vi "IR Laser Diode Controller.vi"() -> ()   [LabVIEW 2014]
doc: "This example shows how to use the TL4000 series driver package with different TL4000 devices (ITC4xxx, LDC4xxx, TED4xxx or CLD1xxx).\n\nNote:\nParts of the Front Panel will be disabled and grayed out if the connected device doesn't suppport the associated functions."
uses:
  <instrlib>/TL4000/TL4000.llb/z_StateMachineTypeDef.ctl
panel:
  out "TEC on?":bool
  out "LD on?":bool
  in  "Config Button":bool
  in  "TEC Button":bool
  in  "LD Button":bool
  in  "Quit Button":bool
  out "PD Optical Power":dbl caption="PD Optical Power [W]" format="%#_4g"
  out "PD Current":dbl caption="PD Current [mA]" format="%#.4g"
  out "Temperature":dbl caption="Temperature [°C]" format="%.2f"
  in  "Temperature Setpoint":dbl=25.0 caption="Temperature [°C]" min=10.0 max=50.0 format="%.2f"
  in  "LD Current Setpoint":dbl caption="LD Current [A]" min=0.0 max=0.48 step=0.1 format="%.4g"
  out "TEC Power":dbl caption="TEC Power [W]" format="%.4f"
  out "TEC Voltage":dbl caption="TEC Voltage [V]" format="%.4f"
  out "TEC Current":dbl caption="TEC Current [A]" format="%.4f"
  out "LD Power":dbl caption="LD electr. Power [W]" format="%.4f"
  out "LD Voltage":dbl caption="LD Voltage [V]" format="%.4f"
  out "LD Current":dbl caption="LD Current [A]" format="%.4f"
  out "Serial Number":string
  out "Device Name":string
  out "Manufacturer Name":string
  out "Firmware Revision":string
  in  "Tab Control":enum32{"Page 1", "Page 2"}(tab)
  in  "error in":errorcluster
  out "error out":errorcluster
  in  "Handle":refnum<visa-resource-name>
  out "State100":T1 caption="States"
  out "user event out":refnum<user-event>
  out "Connected":bool
  in  "Device Type":T2(ring)
  out "Status Bar":string
  # "TL4000 Series Example"
  # "Setpoints:"
  # "Measurement:"
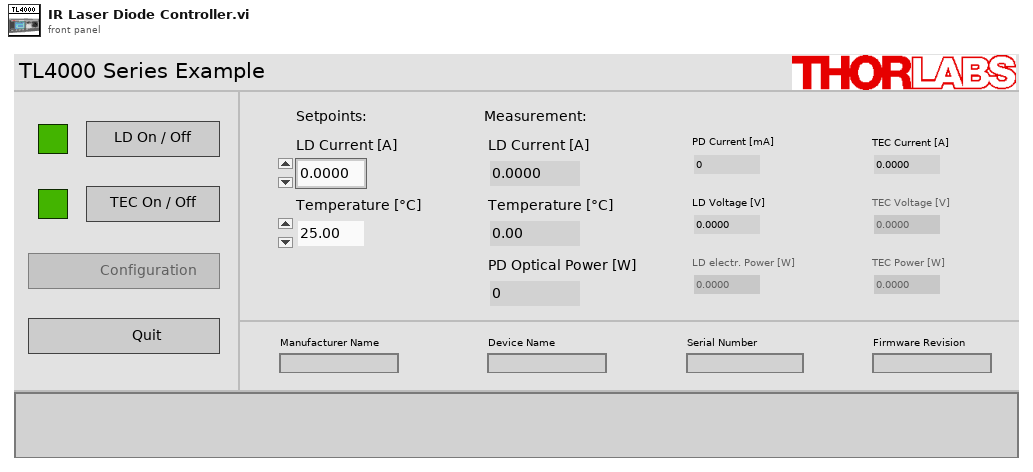
[diagram p1: front panel]
types:
  T1 = typedef "z_StateMachineTypeDef.ctl" = enum16{"Initialize", "1", "2", "3", "4", "5", "6", "7", "8", "9", "10", "15", "20", "25", "30", "35", "40", "45", "50", "55", "59", "60", "65", "70", "75", "76", "77", "78", "79", "80", "85", "90", "91", "92", "93", "94", "95", "96", "97", "98", "99", "100", "105", "110", "120", "130", "140", "150", "160", "170", "180", "190", "200", "205", "210", "215", "220", "230", "240", "245", "250", "255", "260", "270", "280", "290", "300", "310", "313", "315", "318", "320", "330", "340", "350", "360", "370", "380", "390", "400", "410", "420", "430", "440", "450", "460", "470", "480", "490", "500", "510", "520", "523", "525", "528", "530", "540", "550", "560", "570", "580", "590", "600", "605", "610", "620", "630", "640", "650", "660", "670", "680", "690", "700", "710", "720", "730", "740", "750", "760", "770", "780", "790", "800", "810", "820", "830", "840", "850", "860", "870", "880", "890", "900", "910", "920", "930", "940", "950", "960", "970", "980", "990", "1000", "1010", "1020", "1030", "1040", "1050", "1060", "1070", "1080", "1090", "1100", "1110", "1120", "1130", "1140", "1150", "1160", "1170", "1180", "1190", "1200", "1210", "1220", "1230", "1240", "1250", "1260", "1270", "1280", "1290", "1300", "1310", "1320", "1330", "1340", "1350", "1360", "1370", "1380", "1390", "1400", "1410", "1420", "1430", "1440", "1450", "1460", "1470", "1480", "1490", "1500", "Fehler I", "Fehler II", "Fehler III", "Fehler IV", "Fehler V", "Fehler VI", "Fehler VII", "Fehler VIII", "Fehler IX", "Fehler X", "Stop"}
  T2 = enum16{"LDC4000", "CLD1000", "ITC4000", "TED4000"}
  T3 = enum8{"Enabled", "Disabled", "Disabled and Grayed Out"}
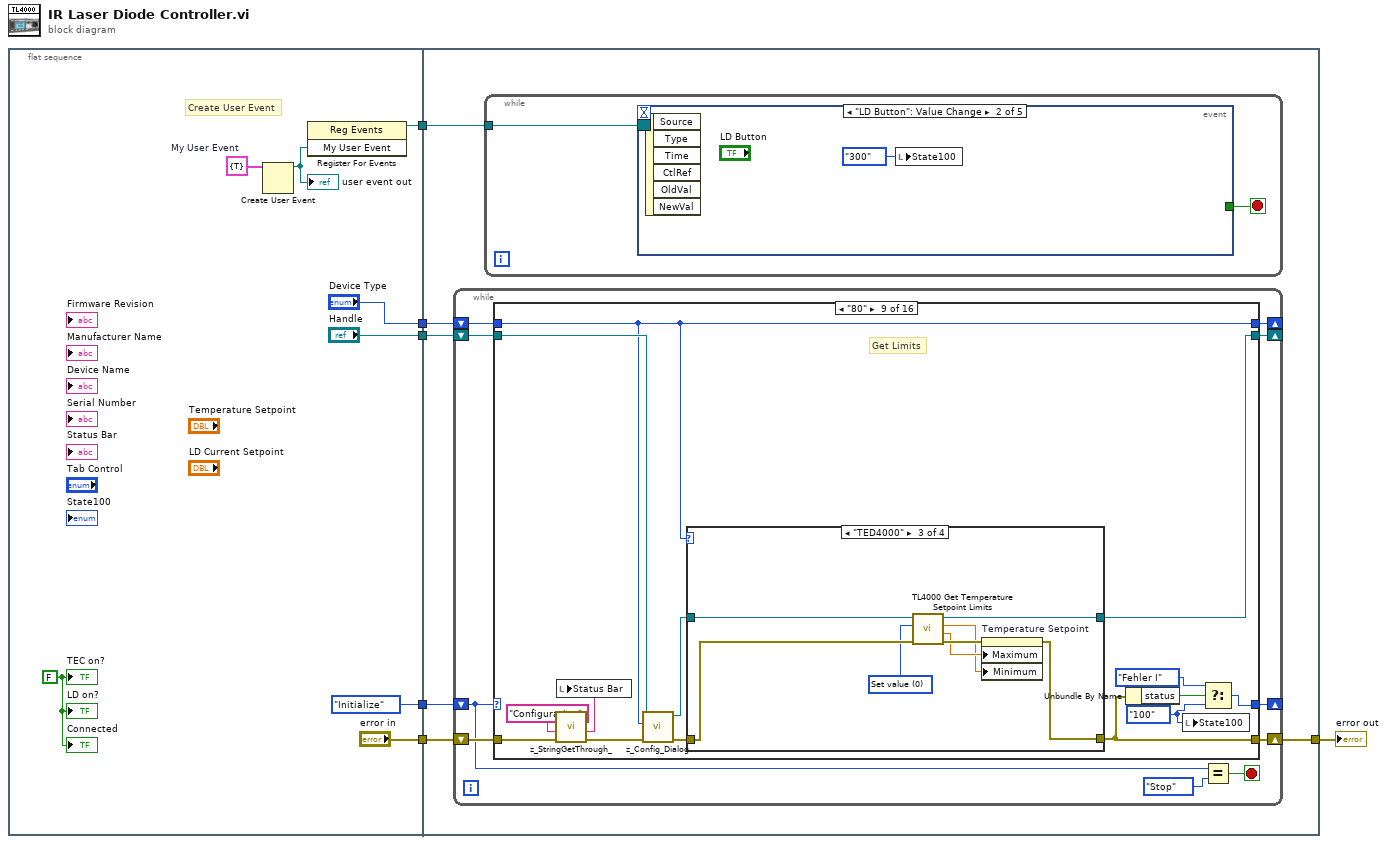
[diagram p0: block diagram]
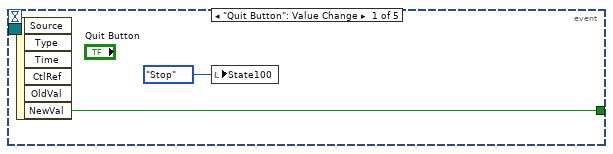
[diagram p2: hidden frame]
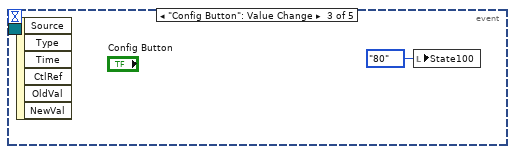
[diagram p3: hidden frame]
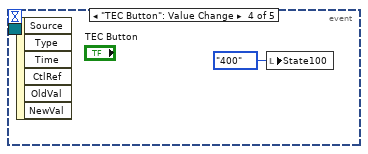
[diagram p4: hidden frame]
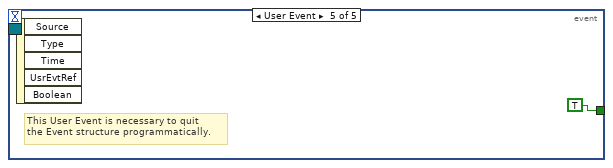
[diagram p5: hidden frame]
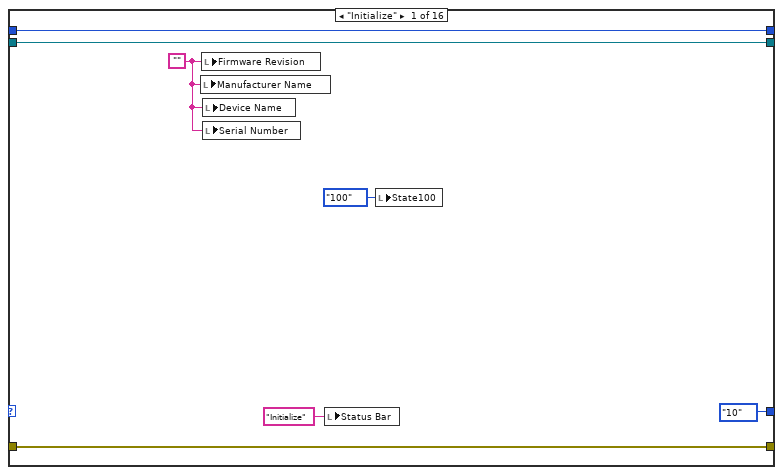
[diagram p6: hidden frame]
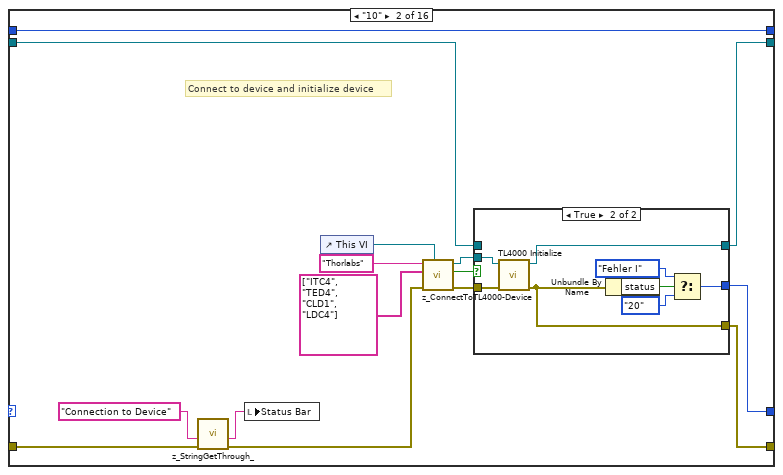
[diagram p7: hidden frame]
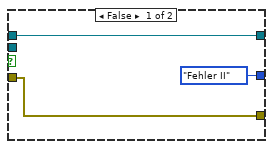
[diagram p8: hidden frame]
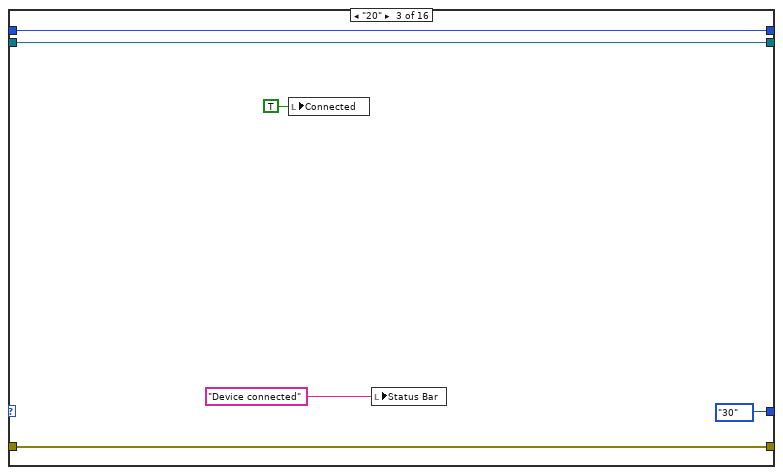
[diagram p9: hidden frame]
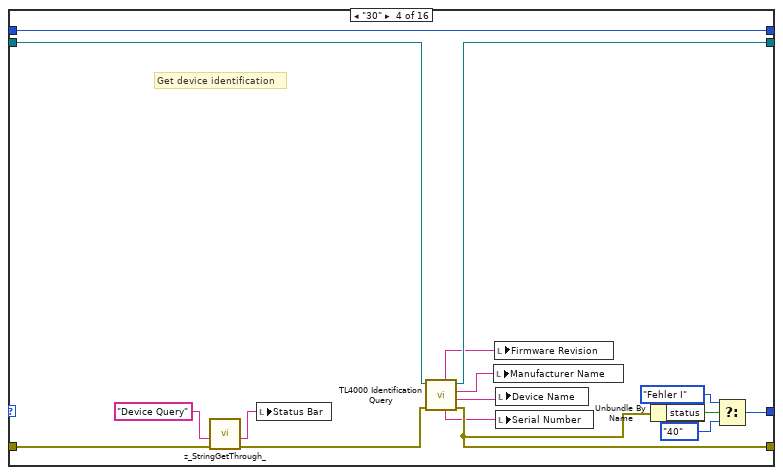
[diagram p10: hidden frame]
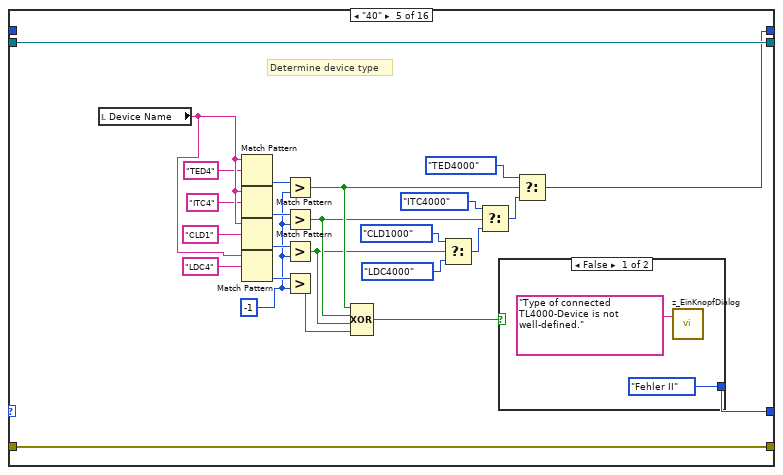
[diagram p11: hidden frame]
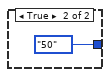
[diagram p12: hidden frame]
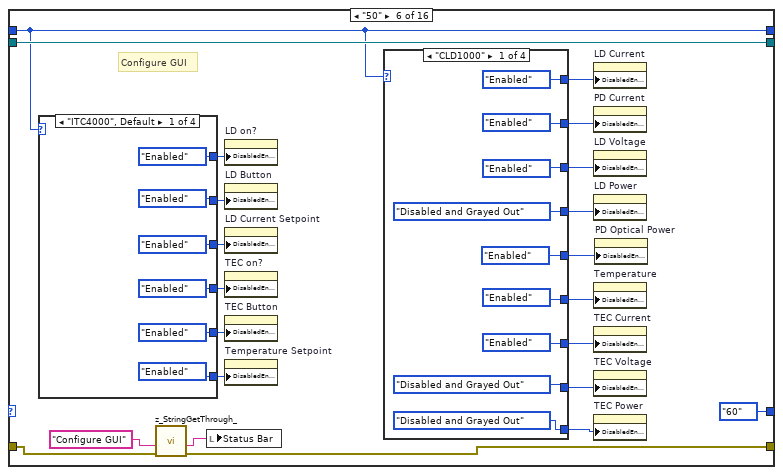
[diagram p13: hidden frame]
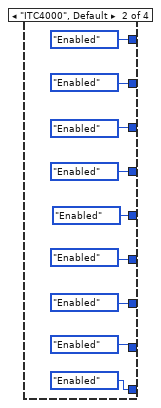
[diagram p14: hidden frame]
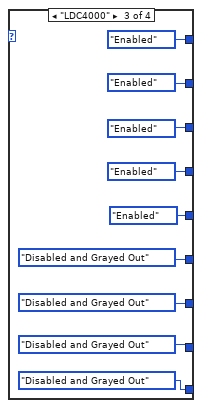
[diagram p15: hidden frame]
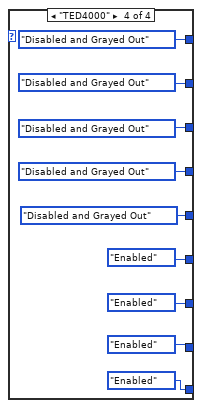
[diagram p16: hidden frame]
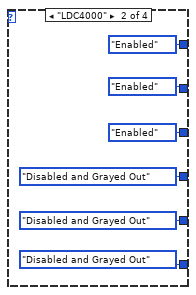
[diagram p17: hidden frame]
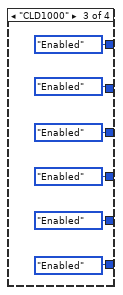
[diagram p18: hidden frame]
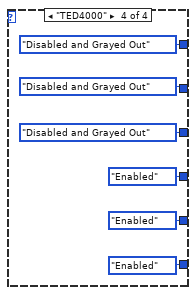
[diagram p19: hidden frame]
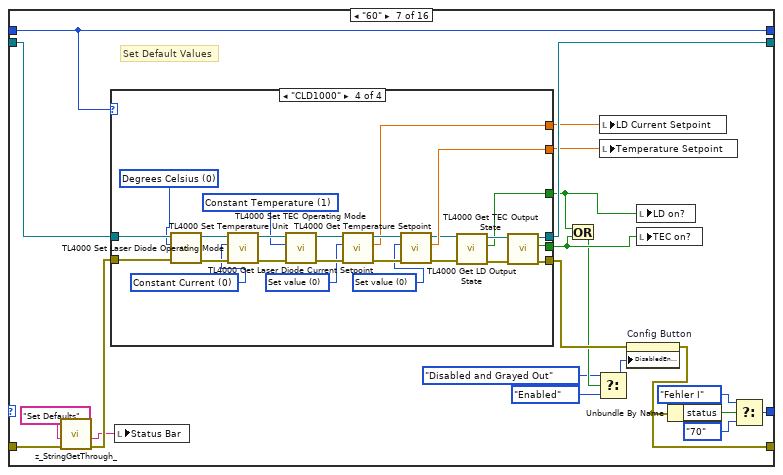
[diagram p20: hidden frame]
diagram:
  n1 = flat-sequence {
    tunnel: ["error in"] -> w6
    tunnel: ["Handle"] -> w4
    tunnel: ["Device Type"] -> w3
    tunnel: [z_StateMachineTypeDef."Initialize" ("States")] -> w2
    tunnel: [w8] -> w1
    tunnel: w6 -> [w20]
    tunnel: [w19] -> w5
    tunnel: w4 -> [w18]
    tunnel: w3 -> [w17]
    tunnel: w2 -> [w16]
    tunnel: w1 -> [w15]
    frame #0 {
      w10 = FALSE ("TEC on?")
      w14 = cluster{"Boolean":bool} {"Boolean"=TRUE}  # My User Event
      # "Create User Event"
      n2 = Create User Event(user event datatype=w14) -> (user event=w7:refnum<user-event>)  [unwired: 1 in, 1 out]
      "user event out" <- w7
      n3 = register-events(w7) -> (reference out=w8:refnum<event-registration>)  [unwired: 2 in, 1 out]
      "Connected" <- w10
      "TEC on?" <- w10
      "LD on?" <- w10
    }
    frame #1 {
      n4 = while {
        shift-right: [w38] -> _
        shift-left: w16 -> [w29]
        shift-right: [w34] -> w19
        shift-left: w20 -> [w35]
        shift-right: [w32] -> _
        shift-left: w18 -> [w33]
        shift-right: [w30] -> _
        shift-left: w17 -> [w31]
        stop <- w36 stop-if-true
        n5 = case shown="\"80\"" w29 {
          tunnel: [z_StateMachineTypeDef."10" ("States") w55 z_StateMachineTypeDef."30" ("States") w90 w101 z_StateMachineTypeDef."60" ("States") w224 w314 w472 z_StateMachineTypeDef."200" ("States") w540 w674 w693 z_StateMachineTypeDef."Fehler II" ("States") z_StateMachineTypeDef."Stop" ("States") z_StateMachineTypeDef."Stop" ("States")] -> w38
          tunnel: w35 -> [w42 w51 w75 w87 w102 w134 w215 w306 w462 w517 w529 w670 w690 w697 w706 w713]
          tunnel: [w42 w54 w75 w85 w102 w133 w210 w310 w467 w517 w537 w667 w678 w703 w706 w712] -> w34
          tunnel: w33 -> [w41 w53 w74 w84 w118 w142 w220 w309 w469 w518 w539 w671 w691 w701 w707 w716]
          tunnel: [w41 w52 w74 w83 w118 w142 w219 w308 w465 w518 w538 w672 w686 w702 w707 w716] -> w32
          tunnel: w31 -> [w39 w47 w72 w78 _ w131 w216 w307 w464 w514 w526 w665 w685 w698 w705 w711]
          tunnel: [w39 w47 w72 w78 w94 w131 w216 w307 w464 w514 w526 w665 w685 w698 w705 w711] -> w30
          frame "Initialize" {
            w43 = ""
            n6 = local write "Manufacturer Name"(w43) -> ()
            n7 = local write "Firmware Revision"(w43) -> ()
            n8 = local write "Device Name"(w43) -> ()
            n9 = local write "Serial Number"(w43) -> ()
            n10 = local write "Status Bar"("Initialize" ("Statuszeile")) -> ()
            n11 = local write "State100"(z_StateMachineTypeDef."100" ("State100")) -> ()
          }
          frame "10" {
            # "Connect to device and initialize device"
            n12 = call <instrlib>:"z_StringGetThrough_.vi"("Error In"=w51, "String In"="Connection to Device") -> ("Error Out"=w50:errorcluster, "String Out"=w49:string)  [unwired: 8 in]
            n13 = local write "Status Bar"(w49) -> ()
            n14 = control-ref of="This VI"() -> (w59:refnum<vi>)
            n15 = call <instrlib>:"z_ConnectToTL4000-Device.vi"("VI reference"=w59, "error in"=w50, "Models"=string[] ["ITC4", "TED4", "CLD1", "LDC4"], "Manufacturer"="Thorlabs") -> ("error out"=w56:errorcluster, "FoundUSB"=w58:bool, "USB Ref"=w57:refnum<visa-resource-name>)  [unwired: 5 in]
            n16 = case shown="True" w58 {
              tunnel: w57 -> [_ w65]
              tunnel: w56 -> [w62 w67]
              tunnel: [z_StateMachineTypeDef."Fehler II" ("f") w68] -> w55
              tunnel: [w62 w66] -> w54
              tunnel: [w63 w64] -> w52
              tunnel: w53 -> [w63 _]
              frame False {
              }
              frame True {
                n17 = call <instrlib>:"TL4000 Initialize.vi"("error in (no error)"=w67, "resource name"=w65) -> ("error out"=w66:errorcluster, "instrument handle out"=w64:refnum<visa-resource-name>)  [unwired: 8 in]
                n18 = Unbundle By Name(w66) -> ("status"=w69:bool)
                n19 = Select(t=z_StateMachineTypeDef."Fehler I" ("States"), s=w69, f=z_StateMachineTypeDef."20") -> (s? t:f=w68:T1)
              }
            }
          }
          frame "20" {
            n20 = local write "Connected"(TRUE ("Connected")) -> ()
            n21 = local write "Status Bar"("Device connected" ("String In")) -> ()
          }
          frame "30" {
            # "Get device identification"
            n22 = call <instrlib>:"z_StringGetThrough_.vi"("Error In"=w87, "String In"="Device Query") -> ("Error Out"=w86:errorcluster, "String Out"=w89:string)  [unwired: 8 in]
            n23 = local write "Status Bar"(w89) -> ()
            n24 = call <instrlib>:"TL4000 Identification Query.vi"("error in (no error)"=w86, "instrument handle"=w84) -> ("error out"=w85:errorcluster, "Device Name"=w80:string, "Manufacturer Name"=w81:string, "instrument handle out"=w83:refnum<visa-resource-name>, "Serial Number"=w79:string, "Firmware Revision"=w82:string)  [unwired: 4 in]
            n25 = local write "Manufacturer Name"(w81) -> ()
            n26 = local write "Firmware Revision"(w82) -> ()
            n27 = local write "Device Name"(w80) -> ()
            n28 = local write "Serial Number"(w79) -> ()
            n29 = Unbundle By Name(w85) -> ("status"=w91:bool)
            n30 = Select(t=z_StateMachineTypeDef."Fehler I" ("States"), s=w91, f=z_StateMachineTypeDef."40") -> (s? t:f=w90:T1)
          }
          frame "40" {
            w108 = -1 ("y")
            # "Determine device type"
            n31 = local read "Device Name"() -> (w117:string)
            n32 = Match Pattern(string=w117, regular expression="TED4") -> (offset past match=w112:i32)  [unwired: 1 in, 3 out]
            n33 = Match Pattern(string=w117, regular expression="ITC4") -> (offset past match=w111:i32)  [unwired: 1 in, 3 out]
            n34 = Match Pattern(string=w117, regular expression="CLD1") -> (offset past match=w110:i32)  [unwired: 1 in, 3 out]
            n35 = Match Pattern(string=w117, regular expression="LDC4") -> (offset past match=w109:i32)  [unwired: 1 in, 3 out]
            n36 = Greater?(x=w112, y=w108) -> (0:w107:bool)
            n37 = Greater?(x=w111, y=w108) -> (0:w106:bool)
            n38 = Greater?(x=w110, y=w108) -> (0:w105:bool)
            n39 = Greater?(x=w109, y=w108) -> (0:w104:bool)
            n40 = Compound Arithmetic op=XOR(w107, w106, w105, w104) -> (w103:bool)
            n41 = Select(t=T2."CLD1000" ("Device_Type"), s=w105, f=T2."LDC4000" ("Device_Type")) -> (s? t:f=w95:T2)
            n42 = Select(t=T2."ITC4000" ("Device_Type"), s=w106, f=w95) -> (s? t:f=w99:T2)
            n43 = case shown="False" w103 {
              tunnel: [z_StateMachineTypeDef."Fehler II" ("States") z_StateMachineTypeDef."50" ("f")] -> w101
              frame False {
                n44 = call <instrlib>:"z_EinKnopfDialog.vi"("Message"="Type of connected TL4000-Device is not well-defined.") -> ()  [unwired: 1 in, 1 out]
              }
              frame True {
              }
            }
            n45 = Select(t=T2."TED4000" ("Device_Type"), s=w107, f=w99) -> (s? t:f=w94:T2)
          }
          frame "50" {
            # "Configure GUI"
            n46 = case shown="\"ITC4000\", Default" w131 {
              tunnel: [T3."Enabled" ("Disabled") T3."Enabled" ("Disabled") T3."Enabled" ("Disabled") T3."Disabled and Grayed Out" ("Disabled")] -> w141
              tunnel: [T3."Enabled" ("Disabled") T3."Enabled" ("Disabled") T3."Enabled" ("Disabled") T3."Disabled and Grayed Out" ("Disabled")] -> w140
              tunnel: [T3."Enabled" ("Disabled") T3."Enabled" ("Disabled") T3."Enabled" ("Disabled") T3."Disabled and Grayed Out" ("Disabled")] -> w139
              tunnel: [T3."Enabled" ("Disabled") T3."Disabled and Grayed Out" ("Disabled") T3."Enabled" ("Disabled") T3."Enabled" ("Disabled")] -> w138
              tunnel: [T3."Enabled" ("Disabled") T3."Disabled and Grayed Out" ("Disabled") T3."Enabled" ("Disabled") T3."Enabled" ("Disabled")] -> w137
              tunnel: [T3."Enabled" ("Disabled") T3."Disabled and Grayed Out" ("Disabled") T3."Enabled" ("Disabled") T3."Enabled" ("Disabled")] -> w136
              frame "ITC4000", Default {
              }
              frame "LDC4000" {
              }
              frame "CLD1000" {
              }
              frame "TED4000" {
              }
            }
            n47 = call <instrlib>:"z_StringGetThrough_.vi"("Error In"=w134, "String In"="Configure GUI") -> ("Error Out"=w133:errorcluster, "String Out"=w132:string)  [unwired: 8 in]
            n48 = local write "Status Bar"(w132) -> ()
            n49 = property on="LD on?" class="Bool (strict)"("DisabledEnum"=w141) -> ()  [unwired: 2 in, 2 out]
            n50 = property on="LD Button" class="Bool"("DisabledEnum"=w140) -> ()  [unwired: 2 in, 2 out]
            n51 = property on="LD Current Setpoint" class="DigNum (strict)"("DisabledEnum"=w139) -> ()  [unwired: 2 in, 2 out]
            n52 = property on="TEC on?" class="Bool (strict)"("DisabledEnum"=w138) -> ()  [unwired: 2 in, 2 out]
            n53 = property on="TEC Button" class="Bool"("DisabledEnum"=w137) -> ()  [unwired: 2 in, 2 out]
            n54 = property on="Temperature Setpoint" class="DigNum (strict)"("DisabledEnum"=w136) -> ()  [unwired: 2 in, 2 out]
            n55 = case shown="\"CLD1000\"" w131 {
              tunnel: [T3."Enabled" ("Disabled") T3."Enabled" ("Disabled") T3."Enabled" ("Disabled") T3."Disabled and Grayed Out" ("Disabled")] -> w123
              tunnel: [T3."Enabled" ("Disabled") T3."Enabled" ("Disabled") T3."Enabled" ("Disabled") T3."Disabled and Grayed Out" ("Disabled")] -> w124
              tunnel: [T3."Disabled and Grayed Out" ("Disabled") T3."Enabled" ("Disabled") T3."Enabled" ("Disabled") T3."Disabled and Grayed Out" ("Disabled")] -> w125
              tunnel: [T3."Enabled" ("Disabled") T3."Enabled" ("Disabled") T3."Disabled and Grayed Out" ("Disabled") T3."Enabled" ("Disabled")] -> w126
              tunnel: [T3."Enabled" ("Disabled") T3."Enabled" ("Disabled") T3."Disabled and Grayed Out" ("Disabled") T3."Enabled" ("Disabled")] -> w127
              tunnel: [T3."Disabled and Grayed Out" ("Disabled") T3."Enabled" ("Disabled") T3."Disabled and Grayed Out" ("Disabled") T3."Enabled" ("Disabled")] -> w128
              tunnel: [T3."Disabled and Grayed Out" ("Disabled") T3."Enabled" ("Disabled") T3."Disabled and Grayed Out" ("Disabled") T3."Enabled" ("Disabled")] -> w130
              tunnel: [T3."Enabled" ("Disabled") T3."Enabled" ("Disabled") T3."Enabled" ("Disabled") T3."Disabled and Grayed Out" ("Disabled")] -> w129
              tunnel: [T3."Enabled" ("Disabled") T3."Enabled" ("Disabled") T3."Enabled" ("Disabled") T3."Disabled and Grayed Out" ("Disabled")] -> w122
              frame "CLD1000" {
              }
              frame "ITC4000", Default {
              }
              frame "LDC4000" {
              }
              frame "TED4000" {
              }
            }
            n56 = property on="LD Current" class="DigNum (strict)"("DisabledEnum"=w129) -> ()  [unwired: 2 in, 2 out]
            n57 = property on="PD Current" class="DigNum (strict)"("DisabledEnum"=w123) -> ()  [unwired: 2 in, 2 out]
            n58 = property on="LD Voltage" class="DigNum (strict)"("DisabledEnum"=w124) -> ()  [unwired: 2 in, 2 out]
            n59 = property on="LD Power" class="DigNum (strict)"("DisabledEnum"=w125) -> ()  [unwired: 2 in, 2 out]
            n60 = property on="Temperature" class="DigNum (strict)"("DisabledEnum"=w126) -> ()  [unwired: 2 in, 2 out]
            n61 = property on="TEC Current" class="DigNum (strict)"("DisabledEnum"=w127) -> ()  [unwired: 2 in, 2 out]
            n62 = property on="TEC Voltage" class="DigNum (strict)"("DisabledEnum"=w128) -> ()  [unwired: 2 in, 2 out]
            n63 = property on="TEC Power" class="DigNum (strict)"("DisabledEnum"=w130) -> ()  [unwired: 2 in, 2 out]
            n64 = property on="PD Optical Power" class="DigNum (strict)"("DisabledEnum"=w122) -> ()  [unwired: 2 in, 2 out]
          }
          frame "60" {
            # "Set Default Values"
            n65 = call <instrlib>:"z_StringGetThrough_.vi"("Error In"=w215, "String In"="Set Defaults") -> ("Error Out"=w214:errorcluster, "String Out"=w212:string)  [unwired: 8 in]
            n66 = case shown="\"CLD1000\"" w216 {
              tunnel: w214 -> [w249 w260 w280 w305]
              tunnel: [w232 w254 w276 w288] -> w211
              tunnel: w220 -> [w244 w261 w279 w300]
              tunnel: [w233 w255 w277 w289] -> w219
              tunnel: [w239 w263 0.0 ("Laser Diode Current Setpoint") w295] -> w218
              tunnel: [w238 0.0 ("Temperature Setpoint") w278 w294] -> w217
              tunnel: [w231 FALSE ("TEC Output") w275 w287] -> w208
              tunnel: [w230 w262 FALSE ("LD Output") w286] -> w209
              frame "ITC4000", Default {
                w225 = i16 0 items=["Set value", "Minimum value", "Maximum value"] ("Attribute (Set value)")
                w226 = i16 0 items=["Set value", "Minimum value", "Maximum value"] ("Attribute (Set value)")
                w227 = i16 1 items=["Constant Temperature"=1, "Current Source"=0] ("TEC Operating Mode (Constant Temperature)")
                w228 = i16 0 items=["Constant Current", "Constant Power"] ("Laser Diode Operating Mode (Constant Current)")
                w229 = i16 0 items=["Degrees Celsius", "Kelvin", "Degrees Fahrenheit"] ("Temperature Unit (Degrees Celsius)")
                n67 = call <instrlib>:"TL4000 Set Temperature Unit.vi"("error in (no error)"=w249, "Temperature Unit (Degrees Celsius)"=w229, "instrument handle"=w244) -> ("error out"=w248:errorcluster, "instrument handle out"=w243:refnum<visa-resource-name>)  [unwired: 7 in]
                n68 = call <instrlib>:"TL4000 Set Laser Diode Operating Mode.vi"("error in (no error)"=w248, "Laser Diode Operating Mode (Constant Current)"=w228, "instrument handle"=w243) -> ("error out"=w247:errorcluster, "instrument handle out"=w242:refnum<visa-resource-name>)  [unwired: 7 in]
                n69 = call <instrlib>:"TL4000 Set TEC Operating Mode.vi"("error in (no error)"=w247, "TEC Operating Mode (Constant Temperature)"=w227, "instrument handle"=w242) -> ("error out"=w246:errorcluster, "instrument handle out"=w241:refnum<visa-resource-name>)  [unwired: 7 in]
                n70 = call <instrlib>:"TL4000 Get Laser Diode Current Setpoint.vi"("error in (no error)"=w246, "Attribute (Set value)"=w226, "instrument handle"=w241) -> ("error out"=w245:errorcluster, "Laser Diode Current Setpoint"=w239:dbl, "instrument handle out"=w240:refnum<visa-resource-name>)  [unwired: 6 in]
                n71 = call <instrlib>:"TL4000 Get Temperature Setpoint.vi"("error in (no error)"=w245, "Attribute (Set value)"=w225, "instrument handle"=w240) -> ("error out"=w236:errorcluster, "Temperature Setpoint"=w238:dbl, "instrument handle out"=w237:refnum<visa-resource-name>)  [unwired: 6 in]
                n72 = call <instrlib>:"TL4000 Get LD Output State.vi"("error in (no error)"=w236, "instrument handle"=w237) -> ("error out"=w234:errorcluster, "LD Output"=w230:bool, "instrument handle out"=w235:refnum<visa-resource-name>)  [unwired: 7 in]
                n73 = call <instrlib>:"TL4000 Get TEC Output State.vi"("error in (no error)"=w234, "instrument handle"=w235) -> ("error out"=w232:errorcluster, "TEC Output"=w231:bool, "instrument handle out"=w233:refnum<visa-resource-name>)  [unwired: 7 in]
              }
              frame "LDC4000" {
                w250 = i16 0 items=["Set value", "Minimum value", "Maximum value"] ("Attribute (Set value)")
                w251 = i16 0 items=["Constant Current", "Constant Power"] ("Laser Diode Operating Mode (Constant Current)")
                n74 = call <instrlib>:"TL4000 Set Laser Diode Operating Mode.vi"("error in (no error)"=w260, "Laser Diode Operating Mode (Constant Current)"=w251, "instrument handle"=w261) -> ("error out"=w258:errorcluster, "instrument handle out"=w259:refnum<visa-resource-name>)  [unwired: 7 in]
                n75 = call <instrlib>:"TL4000 Get Laser Diode Current Setpoint.vi"("error in (no error)"=w258, "Attribute (Set value)"=w250, "instrument handle"=w259) -> ("error out"=w257:errorcluster, "Laser Diode Current Setpoint"=w263:dbl, "instrument handle out"=w256:refnum<visa-resource-name>)  [unwired: 6 in]
                n76 = call <instrlib>:"TL4000 Get LD Output State.vi"("error in (no error)"=w257, "instrument handle"=w256) -> ("error out"=w254:errorcluster, "LD Output"=w262:bool, "instrument handle out"=w255:refnum<visa-resource-name>)  [unwired: 7 in]
              }
              frame "TED4000" {
                w264 = i16 0 items=["Set value", "Minimum value", "Maximum value"] ("Attribute (Set value)")
                w265 = i16 1 items=["Constant Temperature"=1, "Current Source"=0] ("TEC Operating Mode (Constant Temperature)")
                w266 = i16 0 items=["Degrees Celsius", "Kelvin", "Degrees Fahrenheit"] ("Temperature Unit (Degrees Celsius)")
                n77 = call <instrlib>:"TL4000 Set Temperature Unit.vi"("error in (no error)"=w280, "Temperature Unit (Degrees Celsius)"=w266, "instrument handle"=w279) -> ("error out"=w268:errorcluster, "instrument handle out"=w269:refnum<visa-resource-name>)  [unwired: 7 in]
                n78 = call <instrlib>:"TL4000 Set TEC Operating Mode.vi"("error in (no error)"=w268, "TEC Operating Mode (Constant Temperature)"=w265, "instrument handle"=w269) -> ("error out"=w270:errorcluster, "instrument handle out"=w271:refnum<visa-resource-name>)  [unwired: 7 in]
                n79 = call <instrlib>:"TL4000 Get Temperature Setpoint.vi"("error in (no error)"=w270, "Attribute (Set value)"=w264, "instrument handle"=w271) -> ("error out"=w272:errorcluster, "Temperature Setpoint"=w278:dbl, "instrument handle out"=w273:refnum<visa-resource-name>)  [unwired: 6 in]
                n80 = call <instrlib>:"TL4000 Get TEC Output State.vi"("error in (no error)"=w272, "instrument handle"=w273) -> ("error out"=w276:errorcluster, "TEC Output"=w275:bool, "instrument handle out"=w277:refnum<visa-resource-name>)  [unwired: 7 in]
              }
              frame "CLD1000" {
                w281 = i16 0 items=["Set value", "Minimum value", "Maximum value"] ("Attribute (Set value)")
                w282 = i16 0 items=["Set value", "Minimum value", "Maximum value"] ("Attribute (Set value)")
                w283 = i16 1 items=["Constant Temperature"=1, "Current Source"=0] ("TEC Operating Mode (Constant Temperature)")
                w284 = i16 0 items=["Constant Current", "Constant Power"] ("Laser Diode Operating Mode (Constant Current)")
                w285 = i16 0 items=["Degrees Celsius", "Kelvin", "Degrees Fahrenheit"] ("Temperature Unit (Degrees Celsius)")
                n81 = call <instrlib>:"TL4000 Set Temperature Unit.vi"("error in (no error)"=w305, "Temperature Unit (Degrees Celsius)"=w285, "instrument handle"=w300) -> ("error out"=w304:errorcluster, "instrument handle out"=w299:refnum<visa-resource-name>)  [unwired: 7 in]
                n82 = call <instrlib>:"TL4000 Set Laser Diode Operating Mode.vi"("error in (no error)"=w304, "Laser Diode Operating Mode (Constant Current)"=w284, "instrument handle"=w299) -> ("error out"=w303:errorcluster, "instrument handle out"=w298:refnum<visa-resource-name>)  [unwired: 7 in]
                n83 = call <instrlib>:"TL4000 Set TEC Operating Mode.vi"("error in (no error)"=w303, "TEC Operating Mode (Constant Temperature)"=w283, "instrument handle"=w298) -> ("error out"=w302:errorcluster, "instrument handle out"=w297:refnum<visa-resource-name>)  [unwired: 7 in]
                n84 = call <instrlib>:"TL4000 Get Laser Diode Current Setpoint.vi"("error in (no error)"=w302, "Attribute (Set value)"=w282, "instrument handle"=w297) -> ("error out"=w301:errorcluster, "Laser Diode Current Setpoint"=w295:dbl, "instrument handle out"=w296:refnum<visa-resource-name>)  [unwired: 6 in]
                n85 = call <instrlib>:"TL4000 Get Temperature Setpoint.vi"("error in (no error)"=w301, "Attribute (Set value)"=w281, "instrument handle"=w296) -> ("error out"=w292:errorcluster, "Temperature Setpoint"=w294:dbl, "instrument handle out"=w293:refnum<visa-resource-name>)  [unwired: 6 in]
                n86 = call <instrlib>:"TL4000 Get LD Output State.vi"("error in (no error)"=w292, "instrument handle"=w293) -> ("error out"=w290:errorcluster, "LD Output"=w286:bool, "instrument handle out"=w291:refnum<visa-resource-name>)  [unwired: 7 in]
                n87 = call <instrlib>:"TL4000 Get TEC Output State.vi"("error in (no error)"=w290, "instrument handle"=w291) -> ("error out"=w288:errorcluster, "TEC Output"=w287:bool, "instrument handle out"=w289:refnum<visa-resource-name>)  [unwired: 7 in]
              }
            }
            n88 = local write "Status Bar"(w212) -> ()
            n89 = Or(x=w209, y=w208) -> (x .or. y?=w207:bool)
            n90 = Select(t=T3."Disabled and Grayed Out" ("Disabled"), s=w207, f=T3."Enabled" ("Disabled")) -> (s? t:f=w206:T3)
            n91 = local write "LD Current Setpoint"(w218) -> ()
            n92 = local write "Temperature Setpoint"(w217) -> ()
            n93 = property on="Config Button" class="Bool"(error in=w211, "DisabledEnum"=w206) -> (error out=w210:errorcluster)  [unwired: 1 in, 1 out]
            n94 = local write "LD on?"(w209) -> ()
            n95 = local write "TEC on?"(w208) -> ()
            n96 = Unbundle By Name(w210) -> ("status"=w221:bool)
            n97 = Select(t=z_StateMachineTypeDef."Fehler I" ("States"), s=w221, f=z_StateMachineTypeDef."70" ("States")) -> (s? t:f=w224:T1)
          }
          frame "70" {
            # "Set Default Values"
            n98 = case shown="\"ITC4000\", Default" w307 {
              tunnel: w306 -> [w373 w419 w425 w448]
              tunnel: [w335 w389 w423 w440] -> w310
              tunnel: w309 -> [w374 w420 w426 w449]
              tunnel: [w336 w390 w424 w441] -> w308
              frame "ITC4000", Default {
                w315 = i16 0 items=["Disabled (No function)", "Output Enable", "Output Protection"] ("Mode (Disabled (No function))")
                w316 = i16 0 items=["Exponential Method", "Method from Steinhart-Hart"] ("Method (Exponential Method)")
                w318 = i16 0 items=["D-Sub Connector", "Rear Panel BNC"] ("Terminals (D-Sub Connector)")
                w320 = i16 2 items=["Set value", "Minimum value", "Maximum value"] ("Attribute (Set value)")
                w322 = i16 0 items=["Disabled (No function)", "Output Enable", "Output Protection"] ("Mode (Disabled (No function))")
                w324 = i16 2 items=["Set value", "Minimum value", "Maximum value", "Default value"] ("Attribute (Set value)")
                w326 = i16 1 items=["Set value", "Minimum value", "Maximum value", "Default value"] ("Attribute (Set value)")
                w329 = i16 2 items=["Set value", "Minimum value", "Maximum value"] ("Attribute (Set value)")
                w331 = i16 2 items=["Set value", "Minimum value", "Maximum value"] ("Attribute (Set value)")
                w327 = FALSE ("QCW Mode (Off)")
                n99 = call <instrlib>:"TL4000 Get Laser Diode Optical Power Limit.vi"("error in (no error)"=w373, "Attribute (Set value)"=w331, "instrument handle"=w374) -> ("error out"=w371:errorcluster, "Optical Power Limit"=w330:dbl, "instrument handle out"=w372:refnum<visa-resource-name>)  [unwired: 6 in]
                n100 = call <instrlib>:"TL4000 Set Laser Diode Optical Power Limit.vi"("error in (no error)"=w371, "Optical Power Limit (0.0)"=w330, "instrument handle"=w372) -> ("error out"=w369:errorcluster, "instrument handle out"=w370:refnum<visa-resource-name>)  [unwired: 7 in]
                n101 = call <instrlib>:"TL4000 Get Photodiode Current Limit.vi"("error in (no error)"=w369, "Attribute (Set value)"=w329, "instrument handle"=w370) -> ("error out"=w367:errorcluster, "Photodiode Current Limit"=w328:dbl, "instrument handle out"=w368:refnum<visa-resource-name>)  [unwired: 6 in]
                n102 = call <instrlib>:"TL4000 Set Photodiode Current Limit.vi"("error in (no error)"=w367, "Photodiode Current Limit (0.0)"=w328, "instrument handle"=w368) -> ("error out"=w365:errorcluster, "instrument handle out"=w366:refnum<visa-resource-name>)  [unwired: 7 in]
                n103 = call <instrlib>:"TL4000 Switch QCW Mode.vi"("error in (no error)"=w365, "QCW Mode (Off)"=w327, "instrument handle"=w366) -> ("error out"=w363:errorcluster, "instrument handle out"=w364:refnum<visa-resource-name>)  [unwired: 7 in]
                n104 = call <instrlib>:"TL4000 Switch Modulation.vi"("error in (no error)"=w363, "Modulation State (Off)"=w327, "instrument handle"=w364) -> ("error out"=w361:errorcluster, "instrument handle out"=w362:refnum<visa-resource-name>)  [unwired: 7 in]
                n105 = call <instrlib>:"TL4000 Get Output Switch-On Delay.vi"("error in (no error)"=w361, "Attribute (Set value)"=w326, "instrument handle"=w362) -> ("error out"=w359:errorcluster, "Delay"=w325:dbl, "instrument handle out"=w360:refnum<visa-resource-name>)  [unwired: 6 in]
                n106 = call <instrlib>:"TL4000 Set Output Switch-On Delay.vi"("error in (no error)"=w359, "Delay (1.0)"=w325, "instrument handle"=w360) -> ("error out"=w357:errorcluster, "instrument handle out"=w358:refnum<visa-resource-name>)  [unwired: 7 in]
                n107 = call <instrlib>:"TL4000 Get Output Protection Voltage.vi"("error in (no error)"=w357, "Attribute (Set value)"=w324, "instrument handle"=w358) -> ("error out"=w355:errorcluster, "Voltage"=w323:dbl, "instrument handle out"=w356:refnum<visa-resource-name>)  [unwired: 6 in]
                n108 = call <instrlib>:"TL4000 Set Output Protection Voltage.vi"("error in (no error)"=w355, "Voltage (5.0)"=w323, "instrument handle"=w356) -> ("error out"=w354:errorcluster, "instrument handle out"=w353:refnum<visa-resource-name>)  [unwired: 7 in]
                n109 = call <instrlib>:"TL4000 Set LD-Enable Input Mode.vi"("error in (no error)"=w354, "Mode (Disabled (No function))"=w322, "instrument handle"=w353) -> ("error out"=w351:errorcluster, "instrument handle out"=w352:refnum<visa-resource-name>)  [unwired: 7 in]
                n110 = call <instrlib>:"TL4000 Get Photodiode Range.vi"("error in (no error)"=w351, "Attribute (Set value)"=w320, "instrument handle"=w352) -> ("error out"=w349:errorcluster, "Range"=w321:dbl, "instrument handle out"=w350:refnum<visa-resource-name>)  [unwired: 6 in]
                n111 = call <instrlib>:"TL4000 Set Photodiode Range.vi"("error in (no error)"=w349, "Range (0.001)"=w321, "instrument handle"=w350) -> ("error out"=w347:errorcluster, "instrument handle out"=w348:refnum<visa-resource-name>)  [unwired: 7 in]
                n112 = call <instrlib>:"TL4000 Switch Photodiode BIAS.vi"("error in (no error)"=w347, "BIAS State (Off)"=FALSE, "instrument handle"=w348) -> ("error out"=w345:errorcluster, "instrument handle out"=w346:refnum<visa-resource-name>)  [unwired: 7 in]
                n113 = call <instrlib>:"TL4000 Set Photodiode Input Terminals.vi"("error in (no error)"=w345, "Terminals (D-Sub Connector)"=w318, "instrument handle"=w346) -> ("error out"=w343:errorcluster, "instrument handle out"=w344:refnum<visa-resource-name>)  [unwired: 7 in]
                n114 = call <instrlib>:"TL4000 Set Temperature Sensor Offset.vi"("error in (no error)"=w343, "Temperature Offset (0.0)"=0.0, "instrument handle"=w344) -> ("error out"=w341:errorcluster, "instrument handle out"=w342:refnum<visa-resource-name>)  [unwired: 7 in]
                n115 = call <instrlib>:"TL4000 Set Thermistor Method.vi"("error in (no error)"=w341, "Method (Exponential Method)"=w316, "instrument handle"=w342) -> ("error out"=w337:errorcluster, "instrument handle out"=w338:refnum<visa-resource-name>)  [unwired: 7 in]
                n116 = call <instrlib>:"TL4000 Set Thermistor Exponential Parameters.vi"("Beta value (3575.0)"=3575.0, "error in (no error)"=w337, "T0 value (25.0)"=25.0, "R0 value (10.0E3)"=10000.0, "instrument handle"=w338) -> ("error out"=w339:errorcluster, "instrument handle out"=w340:refnum<visa-resource-name>)  [unwired: 5 in]
                n117 = call <instrlib>:"TL4000 Set Temperature Protection Mode.vi"("error in (no error)"=w339, "Mode (Disabled (No function))"=w315, "instrument handle"=w340) -> ("error out"=w335:errorcluster, "instrument handle out"=w336:refnum<visa-resource-name>)  [unwired: 7 in]
              }
              frame "LDC4000" {
                w375 = i16 0 items=["D-Sub Connector", "Rear Panel BNC"] ("Terminals (D-Sub Connector)")
                w378 = i16 2 items=["Set value", "Minimum value", "Maximum value"] ("Attribute (Set value)")
                w379 = i16 0 items=["Disabled (No function)", "Output Enable", "Output Protection"] ("Mode (Disabled (No function))")
                w381 = i16 2 items=["Set value", "Minimum value", "Maximum value", "Default value"] ("Attribute (Set value)")
                w383 = i16 1 items=["Set value", "Minimum value", "Maximum value", "Default value"] ("Attribute (Set value)")
                w386 = i16 2 items=["Set value", "Minimum value", "Maximum value"] ("Attribute (Set value)")
                w388 = i16 2 items=["Set value", "Minimum value", "Maximum value"] ("Attribute (Set value)")
                w384 = FALSE ("QCW Mode (Off)")
                n118 = call <instrlib>:"TL4000 Get Laser Diode Optical Power Limit.vi"("error in (no error)"=w419, "Attribute (Set value)"=w388, "instrument handle"=w420) -> ("error out"=w417:errorcluster, "Optical Power Limit"=w387:dbl, "instrument handle out"=w418:refnum<visa-resource-name>)  [unwired: 6 in]
                n119 = call <instrlib>:"TL4000 Set Laser Diode Optical Power Limit.vi"("error in (no error)"=w417, "Optical Power Limit (0.0)"=w387, "instrument handle"=w418) -> ("error out"=w415:errorcluster, "instrument handle out"=w416:refnum<visa-resource-name>)  [unwired: 7 in]
                n120 = call <instrlib>:"TL4000 Get Photodiode Current Limit.vi"("error in (no error)"=w415, "Attribute (Set value)"=w386, "instrument handle"=w416) -> ("error out"=w413:errorcluster, "Photodiode Current Limit"=w385:dbl, "instrument handle out"=w414:refnum<visa-resource-name>)  [unwired: 6 in]
                n121 = call <instrlib>:"TL4000 Set Photodiode Current Limit.vi"("error in (no error)"=w413, "Photodiode Current Limit (0.0)"=w385, "instrument handle"=w414) -> ("error out"=w411:errorcluster, "instrument handle out"=w412:refnum<visa-resource-name>)  [unwired: 7 in]
                n122 = call <instrlib>:"TL4000 Switch QCW Mode.vi"("error in (no error)"=w411, "QCW Mode (Off)"=w384, "instrument handle"=w412) -> ("error out"=w409:errorcluster, "instrument handle out"=w410:refnum<visa-resource-name>)  [unwired: 7 in]
                n123 = call <instrlib>:"TL4000 Switch Modulation.vi"("error in (no error)"=w409, "Modulation State (Off)"=w384, "instrument handle"=w410) -> ("error out"=w407:errorcluster, "instrument handle out"=w408:refnum<visa-resource-name>)  [unwired: 7 in]
                n124 = call <instrlib>:"TL4000 Get Output Switch-On Delay.vi"("error in (no error)"=w407, "Attribute (Set value)"=w383, "instrument handle"=w408) -> ("error out"=w405:errorcluster, "Delay"=w382:dbl, "instrument handle out"=w406:refnum<visa-resource-name>)  [unwired: 6 in]
                n125 = call <instrlib>:"TL4000 Set Output Switch-On Delay.vi"("error in (no error)"=w405, "Delay (1.0)"=w382, "instrument handle"=w406) -> ("error out"=w403:errorcluster, "instrument handle out"=w404:refnum<visa-resource-name>)  [unwired: 7 in]
                n126 = call <instrlib>:"TL4000 Get Output Protection Voltage.vi"("error in (no error)"=w403, "Attribute (Set value)"=w381, "instrument handle"=w404) -> ("error out"=w401:errorcluster, "Voltage"=w380:dbl, "instrument handle out"=w402:refnum<visa-resource-name>)  [unwired: 6 in]
                n127 = call <instrlib>:"TL4000 Set Output Protection Voltage.vi"("error in (no error)"=w401, "Voltage (5.0)"=w380, "instrument handle"=w402) -> ("error out"=w400:errorcluster, "instrument handle out"=w399:refnum<visa-resource-name>)  [unwired: 7 in]
                n128 = call <instrlib>:"TL4000 Set LD-Enable Input Mode.vi"("error in (no error)"=w400, "Mode (Disabled (No function))"=w379, "instrument handle"=w399) -> ("error out"=w397:errorcluster, "instrument handle out"=w398:refnum<visa-resource-name>)  [unwired: 7 in]
                n129 = call <instrlib>:"TL4000 Get Photodiode Range.vi"("error in (no error)"=w397, "Attribute (Set value)"=w378, "instrument handle"=w398) -> ("error out"=w395:errorcluster, "Range"=w377:dbl, "instrument handle out"=w396:refnum<visa-resource-name>)  [unwired: 6 in]
                n130 = call <instrlib>:"TL4000 Set Photodiode Range.vi"("error in (no error)"=w395, "Range (0.001)"=w377, "instrument handle"=w396) -> ("error out"=w393:errorcluster, "instrument handle out"=w394:refnum<visa-resource-name>)  [unwired: 7 in]
                n131 = call <instrlib>:"TL4000 Switch Photodiode BIAS.vi"("error in (no error)"=w393, "BIAS State (Off)"=FALSE, "instrument handle"=w394) -> ("error out"=w391:errorcluster, "instrument handle out"=w392:refnum<visa-resource-name>)  [unwired: 7 in]
                n132 = call <instrlib>:"TL4000 Set Photodiode Input Terminals.vi"("error in (no error)"=w391, "Terminals (D-Sub Connector)"=w375, "instrument handle"=w392) -> ("error out"=w389:errorcluster, "instrument handle out"=w390:refnum<visa-resource-name>)  [unwired: 7 in]
              }
              frame "TED4000" {
                w421 = i16 0 items=["Exponential Method", "Method from Steinhart-Hart"] ("Method (Exponential Method)")
                n133 = call <instrlib>:"TL4000 Set Temperature Sensor Offset.vi"("error in (no error)"=w425, "Temperature Offset (0.0)"=0.0, "instrument handle"=w426) -> ("error out"=w432:errorcluster, "instrument handle out"=w433:refnum<visa-resource-name>)  [unwired: 7 in]
                n134 = call <instrlib>:"TL4000 Set Thermistor Method.vi"("error in (no error)"=w432, "Method (Exponential Method)"=w421, "instrument handle"=w433) -> ("error out"=w430:errorcluster, "instrument handle out"=w431:refnum<visa-resource-name>)  [unwired: 7 in]
                n135 = call <instrlib>:"TL4000 Set Thermistor Exponential Parameters.vi"("Beta value (3575.0)"=3575.0, "error in (no error)"=w430, "T0 value (25.0)"=25.0, "R0 value (10.0E3)"=10000.0, "instrument handle"=w431) -> ("error out"=w423:errorcluster, "instrument handle out"=w424:refnum<visa-resource-name>)  [unwired: 5 in]
              }
              frame "CLD1000" {
                w434 = i16 0 items=["Disabled (No function)", "Output Enable", "Output Protection"] ("Mode (Disabled (No function))")
                w435 = i16 0 items=["Exponential Method", "Method from Steinhart-Hart"] ("Method (Exponential Method)")
                w438 = i16 2 items=["Set value", "Minimum value", "Maximum value"] ("Attribute (Set value)")
                n136 = call <instrlib>:"TL4000 Switch Modulation.vi"("error in (no error)"=w448, "Modulation State (Off)"=FALSE ("QCW Mode (Off)"), "instrument handle"=w449) -> ("error out"=w446:errorcluster, "instrument handle out"=w447:refnum<visa-resource-name>)  [unwired: 7 in]
                n137 = call <instrlib>:"TL4000 Get Photodiode Range.vi"("error in (no error)"=w446, "Attribute (Set value)"=w438, "instrument handle"=w447) -> ("error out"=w457:errorcluster, "Range"=w437:dbl, "instrument handle out"=w458:refnum<visa-resource-name>)  [unwired: 6 in]
                n138 = call <instrlib>:"TL4000 Set Photodiode Range.vi"("error in (no error)"=w457, "Range (0.001)"=w437, "instrument handle"=w458) -> ("error out"=w455:errorcluster, "instrument handle out"=w456:refnum<visa-resource-name>)  [unwired: 7 in]
                n139 = call <instrlib>:"TL4000 Switch Photodiode BIAS.vi"("error in (no error)"=w455, "BIAS State (Off)"=FALSE, "instrument handle"=w456) -> ("error out"=w444:errorcluster, "instrument handle out"=w445:refnum<visa-resource-name>)  [unwired: 7 in]
                n140 = call <instrlib>:"TL4000 Set Thermistor Method.vi"("error in (no error)"=w444, "Method (Exponential Method)"=w435, "instrument handle"=w445) -> ("error out"=w453:errorcluster, "instrument handle out"=w454:refnum<visa-resource-name>)  [unwired: 7 in]
                n141 = call <instrlib>:"TL4000 Set Thermistor Exponential Parameters.vi"("Beta value (3575.0)"=3575.0, "error in (no error)"=w453, "T0 value (25.0)"=25.0, "R0 value (10.0E3)"=10000.0, "instrument handle"=w454) -> ("error out"=w442:errorcluster, "instrument handle out"=w443:refnum<visa-resource-name>)  [unwired: 5 in]
                n142 = call <instrlib>:"TL4000 Set Temperature Protection Mode.vi"("error in (no error)"=w442, "Mode (Disabled (No function))"=w434, "instrument handle"=w443) -> ("error out"=w440:errorcluster, "instrument handle out"=w441:refnum<visa-resource-name>)  [unwired: 7 in]
              }
            }
            n143 = Unbundle By Name(w310) -> ("status"=w311:bool)
            n144 = Select(t=z_StateMachineTypeDef."Fehler I" ("States"), s=w311, f=z_StateMachineTypeDef."80" ("States")) -> (s? t:f=w314:T1)
          }
          frame "80" {
            w463 = z_StateMachineTypeDef."100" ("States")
            # "Get Limits"
            n145 = call <instrlib>:"z_StringGetThrough_.vi"("Error In"=w462, "String In"="Configuration") -> ("Error Out"=w461:errorcluster, "String Out"=w460:string)  [unwired: 8 in]
            n146 = local write "Status Bar"(w460) -> ()
            n147 = call <instrlib>:"z_Config_Dialog.vi"("Error In"=w461, "Device_Type"=w464, "TE4000 Handle In"=w469) -> ("Error Out"=w468:errorcluster, "TE4000 Handle Out"=w466:refnum<visa-resource-name>)  [unwired: 7 in]
            n148 = case shown="\"TED4000\"" w464 {
              tunnel: w468 -> [w485 w492 w494 w513]
              tunnel: [w477 w487 w498 w505] -> w467
              tunnel: w466 -> [w484 w491 w495 w512]
              tunnel: [w482 w488 w500 w510] -> w465
              frame "ITC4000", Default {
                w473 = i16 0 items=["Set value", "Minimum value", "Maximum value"] ("Attribute (Set value)")
                w474 = i16 0 items=["Set value", "Minimum value", "Maximum value"] ("Attribute (Set value)")
                n149 = call <instrlib>:"TL4000 Get Laser Diode Current Limit.vi"("error in (no error)"=w485, "Attribute (Set value)"=w474, "instrument handle"=w484) -> ("error out"=w481:errorcluster, "Laser Diode Current Limit"=w479:dbl, "instrument handle out"=w483:refnum<visa-resource-name>)  [unwired: 6 in]
                n150 = property on="LD Current Setpoint" class="DigNum (strict)"(error in=w481, "Maximum"=w479) -> (error out=w480:errorcluster)  [unwired: 1 in, 1 out]
                n151 = call <instrlib>:"TL4000 Get Temperature Setpoint Limits.vi"("error in (no error)"=w480, "Attribute (Set value)"=w473, "instrument handle"=w483) -> ("error out"=w478:errorcluster, "Setpoint High Limit"=w476:dbl, "Setpoint Low Limit"=w475:dbl, "instrument handle out"=w482:refnum<visa-resource-name>)  [unwired: 5 in]
                n152 = property on="Temperature Setpoint" class="DigNum (strict)"(error in=w478, "Maximum"=w476, "Minimum"=w475) -> (error out=w477:errorcluster)  [unwired: 1 in, 1 out]
              }
              frame "LDC4000" {
                w486 = i16 0 items=["Set value", "Minimum value", "Maximum value"] ("Attribute (Set value)")
                n153 = call <instrlib>:"TL4000 Get Laser Diode Current Limit.vi"("error in (no error)"=w492, "Attribute (Set value)"=w486, "instrument handle"=w491) -> ("error out"=w490:errorcluster, "Laser Diode Current Limit"=w489:dbl, "instrument handle out"=w488:refnum<visa-resource-name>)  [unwired: 6 in]
                n154 = property on="LD Current Setpoint" class="DigNum (strict)"(error in=w490, "Maximum"=w489) -> (error out=w487:errorcluster)  [unwired: 1 in, 1 out]
              }
              frame "TED4000" {
                w493 = i16 0 items=["Set value", "Minimum value", "Maximum value"] ("Attribute (Set value)")
                n155 = call <instrlib>:"TL4000 Get Temperature Setpoint Limits.vi"("error in (no error)"=w494, "Attribute (Set value)"=w493, "instrument handle"=w495) -> ("error out"=w499:errorcluster, "Setpoint High Limit"=w497:dbl, "Setpoint Low Limit"=w496:dbl, "instrument handle out"=w500:refnum<visa-resource-name>)  [unwired: 5 in]
                n156 = property on="Temperature Setpoint" class="DigNum (strict)"(error in=w499, "Maximum"=w497, "Minimum"=w496) -> (error out=w498:errorcluster)  [unwired: 1 in, 1 out]
              }
              frame "CLD1000" {
                w502 = i16 0 items=["Set value", "Minimum value", "Maximum value"] ("Attribute (Set value)")
                w501 = i16 0 items=["Set value", "Minimum value", "Maximum value"] ("Attribute (Set value)")
                n157 = call <instrlib>:"TL4000 Get Laser Diode Current Limit.vi"("error in (no error)"=w513, "Attribute (Set value)"=w501, "instrument handle"=w512) -> ("error out"=w509:errorcluster, "Laser Diode Current Limit"=w507:dbl, "instrument handle out"=w511:refnum<visa-resource-name>)  [unwired: 6 in]
                n158 = property on="LD Current Setpoint" class="DigNum (strict)"(error in=w509, "Maximum"=w507) -> (error out=w508:errorcluster)  [unwired: 1 in, 1 out]
                n159 = call <instrlib>:"TL4000 Get Temperature Setpoint Limits.vi"("error in (no error)"=w508, "Attribute (Set value)"=w502, "instrument handle"=w511) -> ("error out"=w506:errorcluster, "Setpoint High Limit"=w504:dbl, "Setpoint Low Limit"=w503:dbl, "instrument handle out"=w510:refnum<visa-resource-name>)  [unwired: 5 in]
                n160 = property on="Temperature Setpoint" class="DigNum (strict)"(error in=w506, "Maximum"=w504, "Minimum"=w503) -> (error out=w505:errorcluster)  [unwired: 1 in, 1 out]
              }
            }
            n161 = Unbundle By Name(w467) -> ("status"=w470:bool)
            n162 = local write "State100"(w463) -> ()
            n163 = Select(t=z_StateMachineTypeDef."Fehler I" ("States"), s=w470, f=w463) -> (s? t:f=w472:T1)
          }
          frame "100" {
            n164 = local write "Status Bar"("Default State" ("String In")) -> ()
            n165 = Wait Until Next ms Multiple(millisecond multiple=u32 50) -> ()  [unwired: 1 out]
          }
          frame "200" {
            # "Measurement"
            n166 = local read "Temperature Setpoint"() -> (w527:dbl)
            n167 = local read "LD Current Setpoint"() -> (w530:dbl)
            n168 = case shown="\"TED4000\"" w526 {
              tunnel: w539 -> [w569 w598 w611 w654]
              tunnel: [w553 w584 w614 w633] -> w538
              tunnel: w529 -> [w568 w597 w610 w653]
              tunnel: [w552 w583 w613 w630] -> w537
              tunnel: [w567 w596 0.0 ("Laser Current") w650] -> w536
              tunnel: [w564 w595 0.0 ("Laser Voltage") w647] -> w535
              tunnel: [w563 w594 0.0 ("Power") 0.0 ("Power")] -> w534
              tunnel: [w572 0.0 ("TEC Current") w620 w655] -> w533
              tunnel: [w571 0.0 ("TEC Voltage") w619 0.0 ("TEC Voltage")] -> w532
              tunnel: [w570 0.0 ("TEC Power") w618 0.0 ("TEC Power")] -> w531
              tunnel: w530 -> [w542 w577 _ w625]
              tunnel: w527 -> [w543 _ w599 w626]
              tunnel: [w558 0.0 ("Temperature") w615 w642] -> w525
              tunnel: [w556 w592 0.0 w640] -> w524
              tunnel: [w554 w590 0.0 ("Optical Power Pd") w638] -> w523
              tunnel: [w551 w589 FALSE ("LD Output") w629] -> w521
              tunnel: [w550 FALSE ("TEC Output") w612 w628] -> w520
              frame "ITC4000", Default {
                n169 = call <instrlib>:"TL4000 Set Laser Diode Current Setpoint.vi"("error in (no error)"=w568, "Laser Diode Current Setpoint (0.0)"=w542, "instrument handle"=w569) -> ("error out"=w544:errorcluster, "instrument handle out"=w545:refnum<visa-resource-name>)  [unwired: 7 in]
                n170 = call <instrlib>:"TL4000 Set Temperature Setpoint.vi"("error in (no error)"=w544, "Temperature Setpoint (25.0)"=w543, "instrument handle"=w545) -> ("error out"=w565:errorcluster, "instrument handle out"=w566:refnum<visa-resource-name>)  [unwired: 7 in]
                n171 = call <instrlib>:"TL4000 Measure Laser Diode Multiple Values.vi"("instrument handle"=w566, "error in (no error)"=w565) -> ("Optical Power Pd (0)"=w554:dbl, "instrument handle out"=w561:refnum<visa-resource-name>, "Laser Current"=w567:dbl, "Laser Voltage (0)"=w564:dbl, "Power (0)"=w563:dbl, "Photodiode Current (0)"=w557:dbl, "error out"=w562:errorcluster)  [unwired: 5 in, 2 out]
                n172 = Multiply(x=w557, y=1000.0) -> (x*y=w556:dbl)
                n173 = call <instrlib>:"TL4000 Measure Temperature.vi"("error in (no error)"=w562, "instrument handle"=w561) -> ("error out"=w559:errorcluster, "Temperature"=w558:dbl, "instrument handle out"=w560:refnum<visa-resource-name>)  [unwired: 7 in]
                n174 = call <instrlib>:"TL4000 Measure TEC Current.vi"("error in (no error)"=w559, "instrument handle"=w560) -> ("error out"=w575:errorcluster, "TEC Current"=w572:dbl, "instrument handle out"=w576:refnum<visa-resource-name>)  [unwired: 7 in]
                n175 = call <instrlib>:"TL4000 Measure TEC Voltage.vi"("error in (no error)"=w575, "instrument handle"=w576) -> ("error out"=w573:errorcluster, "TEC Voltage"=w571:dbl, "instrument handle out"=w574:refnum<visa-resource-name>)  [unwired: 7 in]
                n176 = call <instrlib>:"TL4000 Measure TEC Power.vi"("error in (no error)"=w573, "instrument handle"=w574) -> ("error out"=w548:errorcluster, "TEC Power"=w570:dbl, "instrument handle out"=w549:refnum<visa-resource-name>)  [unwired: 7 in]
                n177 = call <instrlib>:"TL4000 Get LD Output State.vi"("error in (no error)"=w548, "instrument handle"=w549) -> ("error out"=w546:errorcluster, "LD Output"=w551:bool, "instrument handle out"=w547:refnum<visa-resource-name>)  [unwired: 7 in]
                n178 = call <instrlib>:"TL4000 Get TEC Output State.vi"("error in (no error)"=w546, "instrument handle"=w547) -> ("error out"=w552:errorcluster, "TEC Output"=w550:bool, "instrument handle out"=w553:refnum<visa-resource-name>)  [unwired: 7 in]
              }
              frame "LDC4000" {
                n179 = call <instrlib>:"TL4000 Set Laser Diode Current Setpoint.vi"("error in (no error)"=w597, "Laser Diode Current Setpoint (0.0)"=w577, "instrument handle"=w598) -> ("error out"=w587:errorcluster, "instrument handle out"=w588:refnum<visa-resource-name>)  [unwired: 7 in]
                n180 = call <instrlib>:"TL4000 Measure Laser Diode Multiple Values.vi"("instrument handle"=w588, "error in (no error)"=w587) -> ("Optical Power Pd (0)"=w590:dbl, "instrument handle out"=w586:refnum<visa-resource-name>, "Laser Current"=w596:dbl, "Laser Voltage (0)"=w595:dbl, "Power (0)"=w594:dbl, "Photodiode Current (0)"=w593:dbl, "error out"=w585:errorcluster)  [unwired: 5 in, 2 out]
                n181 = Multiply(x=w593, y=1000.0) -> (x*y=w592:dbl)
                n182 = call <instrlib>:"TL4000 Get LD Output State.vi"("error in (no error)"=w585, "instrument handle"=w586) -> ("error out"=w583:errorcluster, "LD Output"=w589:bool, "instrument handle out"=w584:refnum<visa-resource-name>)  [unwired: 7 in]
              }
              frame "TED4000" {
                n183 = call <instrlib>:"TL4000 Set Temperature Setpoint.vi"("error in (no error)"=w610, "Temperature Setpoint (25.0)"=w599, "instrument handle"=w611) -> ("error out"=w608:errorcluster, "instrument handle out"=w609:refnum<visa-resource-name>)  [unwired: 7 in]
                n184 = call <instrlib>:"TL4000 Measure Temperature.vi"("error in (no error)"=w608, "instrument handle"=w609) -> ("error out"=w616:errorcluster, "Temperature"=w615:dbl, "instrument handle out"=w617:refnum<visa-resource-name>)  [unwired: 7 in]
                n185 = call <instrlib>:"TL4000 Measure TEC Current.vi"("error in (no error)"=w616, "instrument handle"=w617) -> ("error out"=w623:errorcluster, "TEC Current"=w620:dbl, "instrument handle out"=w624:refnum<visa-resource-name>)  [unwired: 7 in]
                n186 = call <instrlib>:"TL4000 Measure TEC Voltage.vi"("error in (no error)"=w623, "instrument handle"=w624) -> ("error out"=w621:errorcluster, "TEC Voltage"=w619:dbl, "instrument handle out"=w622:refnum<visa-resource-name>)  [unwired: 7 in]
                n187 = call <instrlib>:"TL4000 Measure TEC Power.vi"("error in (no error)"=w621, "instrument handle"=w622) -> ("error out"=w606:errorcluster, "TEC Power"=w618:dbl, "instrument handle out"=w607:refnum<visa-resource-name>)  [unwired: 7 in]
                n188 = call <instrlib>:"TL4000 Get TEC Output State.vi"("error in (no error)"=w606, "instrument handle"=w607) -> ("error out"=w613:errorcluster, "TEC Output"=w612:bool, "instrument handle out"=w614:refnum<visa-resource-name>)  [unwired: 7 in]
              }
              frame "CLD1000" {
                n189 = call <instrlib>:"TL4000 Set Laser Diode Current Setpoint.vi"("error in (no error)"=w653, "Laser Diode Current Setpoint (0.0)"=w625, "instrument handle"=w654) -> ("error out"=w651:errorcluster, "instrument handle out"=w652:refnum<visa-resource-name>)  [unwired: 7 in]
                n190 = call <instrlib>:"TL4000 Set Temperature Setpoint.vi"("error in (no error)"=w651, "Temperature Setpoint (25.0)"=w626, "instrument handle"=w652) -> ("error out"=w648:errorcluster, "instrument handle out"=w649:refnum<visa-resource-name>)  [unwired: 7 in]
                n191 = call <instrlib>:"TL4000 Measure Laser Diode Multiple Values.vi"("instrument handle"=w649, "error in (no error)"=w648) -> ("Optical Power Pd (0)"=w638:dbl, "instrument handle out"=w645:refnum<visa-resource-name>, "Laser Current"=w650:dbl, "Laser Voltage (0)"=w647:dbl, "Photodiode Current (0)"=w641:dbl, "error out"=w646:errorcluster)  [unwired: 5 in, 3 out]
                n192 = Multiply(x=w641, y=1000.0) -> (x*y=w640:dbl)
                n193 = call <instrlib>:"TL4000 Measure Temperature.vi"("error in (no error)"=w646, "instrument handle"=w645) -> ("error out"=w643:errorcluster, "Temperature"=w642:dbl, "instrument handle out"=w644:refnum<visa-resource-name>)  [unwired: 7 in]
                n194 = call <instrlib>:"TL4000 Measure TEC Current.vi"("error in (no error)"=w643, "instrument handle"=w644) -> ("error out"=w632:errorcluster, "TEC Current"=w655:dbl, "instrument handle out"=w635:refnum<visa-resource-name>)  [unwired: 7 in]
                n195 = call <instrlib>:"TL4000 Get LD Output State.vi"("error in (no error)"=w632, "instrument handle"=w635) -> ("error out"=w631:errorcluster, "LD Output"=w629:bool, "instrument handle out"=w634:refnum<visa-resource-name>)  [unwired: 7 in]
                n196 = call <instrlib>:"TL4000 Get TEC Output State.vi"("error in (no error)"=w631, "instrument handle"=w634) -> ("error out"=w630:errorcluster, "TEC Output"=w628:bool, "instrument handle out"=w633:refnum<visa-resource-name>)  [unwired: 7 in]
              }
            }
            "LD Current" <- w536
            "LD Voltage" <- w535
            "LD Power" <- w534
            "TEC Current" <- w533
            "TEC Voltage" <- w532
            "TEC Power" <- w531
            "Temperature" <- w525
            "PD Current" <- w524
            "PD Optical Power" <- w523
            n197 = local write "LD on?"(w521) -> ()
            n198 = local write "TEC on?"(w520) -> ()
            n199 = local read "State100"() -> (w528:T1)
            n200 = Unbundle By Name(w537) -> ("status"=w522:bool)
            n201 = Select(t=z_StateMachineTypeDef."Fehler I" ("States"), s=w522, f=w528) -> (s? t:f=w540:T1)
          }
          frame "300" {
            w668 = z_StateMachineTypeDef."100" ("f")
            # "Switch LD Output"
            n202 = call <instrlib>:"TL4000 Get LD Output State.vi"("error in (no error)"=w670, "instrument handle"=w671) -> ("error out"=w657:errorcluster, "LD Output"=w666:bool, "instrument handle out"=w658:refnum<visa-resource-name>)  [unwired: 7 in]
            n203 = local read "TEC on?"() -> (w660:bool)
            n204 = Not(x=w666) -> (.not. x?=w656:bool)
            n205 = call <instrlib>:"TL4000 Switch LD Output.vi"("error in (no error)"=w657, "LD Output (Off)"=w656, "instrument handle"=w658) -> ("error out"=w664:errorcluster, "instrument handle out"=w672:refnum<visa-resource-name>)  [unwired: 7 in]
            n206 = Or(x=w656, y=w660) -> (x .or. y?=w659:bool)
            n207 = local write "LD on?"(w656) -> ()
            n208 = Select(t=T3."Disabled and Grayed Out" ("Disabled"), s=w659, f=T3."Enabled" ("Disabled")) -> (s? t:f=w663:T3)
            n209 = property on="Config Button" class="Bool"(error in=w664, "DisabledEnum"=w663) -> (error out=w667:errorcluster)  [unwired: 1 in, 1 out]
            n210 = Unbundle By Name(w667) -> ("status"=w669:bool)
            n211 = local write "State100"(w668) -> ()
            n212 = Select(t=z_StateMachineTypeDef."Fehler I" ("States"), s=w669, f=w668) -> (s? t:f=w674:T1)
          }
          frame "400" {
            w683 = z_StateMachineTypeDef."100" ("f")
            # "Switch TEC Output"
            n213 = call <instrlib>:"TL4000 Get TEC Output State.vi"("error in (no error)"=w690, "instrument handle"=w691) -> ("error out"=w687:errorcluster, "TEC Output"=w689:bool, "instrument handle out"=w688:refnum<visa-resource-name>)  [unwired: 7 in]
            n214 = local read "LD on?"() -> (w677:bool)
            n215 = Not(x=w689) -> (.not. x?=w675:bool)
            n216 = Or(x=w675, y=w677) -> (x .or. y?=w676:bool)
            n217 = call <instrlib>:"TL4000 Switch TEC Output.vi"("error in (no error)"=w687, "TEC Output (Off)"=w675, "instrument handle"=w688) -> ("error out"=w679:errorcluster, "instrument handle out"=w686:refnum<visa-resource-name>)  [unwired: 7 in]
            n218 = local write "TEC on?"(w675) -> ()
            n219 = Select(t=T3."Disabled and Grayed Out" ("Disabled"), s=w676, f=T3."Enabled" ("Disabled")) -> (s? t:f=w682:T3)
            n220 = property on="Config Button" class="Bool"(error in=w679, "DisabledEnum"=w682) -> (error out=w678:errorcluster)  [unwired: 1 in, 1 out]
            n221 = Unbundle By Name(w678) -> ("status"=w684:bool)
            n222 = local write "State100"(w683) -> ()
            n223 = Select(t=z_StateMachineTypeDef."Fehler I" ("States"), s=w684, f=w683) -> (s? t:f=w693:T1)
          }
          frame "Fehler I" {
            # "Place the ErrorHandler.vi here\n\nA error message should popup\nin case an error occured."
            n224 = call <instrlib>:"z_StringGetThrough_.vi"("Error In"=w697, "String In"="Error!") -> ("Error Out"=w696:errorcluster, "String Out"=w695:string)  [unwired: 8 in]
            n225 = local write "Status Bar"(w695) -> ()
            n226 = Unbundle By Name(w696) -> ("code"=w700:i32)
            n227 = call <instrlib>:"TL4000 Error Message.vi"("error in (no error)"=w696, "Error Code (0)"=w700, "instrument handle"=w701) -> ("error out"=w703:errorcluster, "Error Message"=w699:string, "instrument handle out"=w702:refnum<visa-resource-name>)  [unwired: 6 in]
            n228 = call <instrlib>:"z_EinKnopfDialog.vi"("Message"=w699) -> ()  [unwired: 1 in, 1 out]
          }
          frame "Fehler II" {
            # "Fire User Event"
            n229 = local read "user event out"() -> (w709:refnum<user-event>)
            n230 = Generate User Event(user event=w709, event data cluster=cluster{"Boolean":bool} {"Boolean"=TRUE} ("event data")) -> ()  [unwired: 2 in, 2 out]
          }
          frame "Stop", Default {
            n231 = local read "Connected"() -> (w717:bool)
            n232 = case shown="True" w717 {
              tunnel: w716 -> [_ w719]
              frame False {
              }
              frame True {
                n233 = local write "Connected"(FALSE ("Connected")) -> ()
                n234 = call <instrlib>:"TL4000 Close.vi"("instrument handle"=w719) -> ()  [unwired: 10 in, 1 out]
              }
            }
            n235 = call <instrlib>:"z_StringGetThrough_.vi"("Error In"=w713, "String In"="Program Quit") -> ("Error Out"=w712:errorcluster, "String Out"=w715:string)  [unwired: 8 in]
            n236 = local write "Status Bar"(w715) -> ()
          }
        }
        n237 = Equal?(x=w29, y=z_StateMachineTypeDef."Stop" ("States")) -> (x = y?=w36:bool)
      }
      n238 = while {
        tunnel: w15 -> [w21]
        stop <- w22 stop-if-true
        n239 = event shown="[1] \"LD Button\": Value Change" {
          selector: w21 -> [_ _ _ _ _]
          dyn-events: _ -> [_ _ _ _ _]
          timeout: _ -> [_ _ _ _ _]
          tunnel: [w24 _ _ _ TRUE ("NewVal")] -> w22
          event "Quit Button": Value Change {
            n240 = event-data() -> ("NewVal"=w24:bool)  [unwired: 6 out]
            n241 = local write "State100"(z_StateMachineTypeDef."Stop" ("State100")) -> ()
          }
          event "LD Button": Value Change {
            n242 = event-data() -> ()  [unwired: 7 out]
            n243 = local write "State100"(z_StateMachineTypeDef."300" ("State100")) -> ()
          }
          event "Config Button": Value Change {
            n244 = event-data() -> ()  [unwired: 7 out]
            n245 = local write "State100"(z_StateMachineTypeDef."80" ("State100")) -> ()
          }
          event "TEC Button": Value Change {
            n246 = event-data() -> ()  [unwired: 7 out]
            n247 = local write "State100"(z_StateMachineTypeDef."400" ("State100")) -> ()
          }
          event User Event {
            # "This User Event is necessary to quit\nthe Event structure programmatically."
            n248 = event-data() -> ()  [unwired: 6 out]
          }
        }
      }
    }
  }
  "error out" <- w5
